vi "filter_chebyshev.vi"() -> ()   [LabVIEW 2014]
uses:
  <vilib>/addons/Digital Filter Design/_Objects.llb/DFD Phase Setting.ctl
  <vilib>/addons/Digital Filter Design/Analysis.llb/DFD Plot Freq Response (Linear-Spaced).vi
  <vilib>/addons/Digital Filter Design/NI_DigFilterLicensed.lvlib
panel:
  in  "Ripple":dbl(slide)=1.0 min=1.0 scale=0.0..10.0
  in  "High Cutoff Frequency":dbl(knob)=10.0 min=10.0 scale=0.0..1000.0
  in  "Low Cutoff Frequency":dbl(knob)=1.0 min=1.0 scale=0.0..1000.0
  in  "Scale":bool
  in  "Sampling Rate":dbl=1000.0 min=1000.0
  out "magnitude response":cluster{"f0":dbl, "df":dbl, "values":dbl[]}[](graph)
  out "phase response":cluster{"f0":dbl, "df":dbl, "values":dbl[]}[](graph)
  in  "Order":dbl=1.0 min=1.0
  in  "Filter Type":u16(ring) items=["Lowpass", "Highpass", "Bandpass", "Bandstop"]
  in  "stop":bool
  # "IIR Chebyshev Filters"
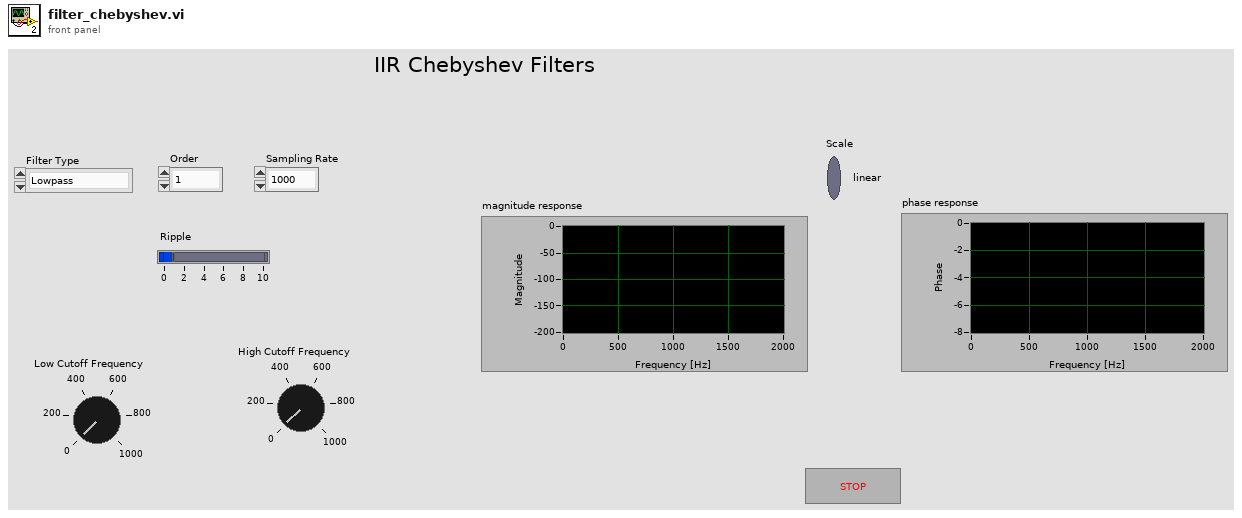
[diagram p1: front panel]
types:
  T1 = typedef "NI_DigFilterLicensed.lvlib/DFD Phase Setting.ctl" = cluster{"unwrap? (F)":bool, "degree? (F)":bool}
  T2 = typedef "NI_DigFilterLicensed.lvlib/DFD Filter Obj.ctl" = cluster{"mSRate_Fs":dbl, "mSRate_Version":string, "mSRate_Comments":string, "mSRate_OrgCoef":T3, "mSRate_CurCoef":T3, "mSRate_Quantized?":bool, "mSRate_QCoef":T3, "mSRate_QSettings":T5[], "mSRate_Order":i32, "mSRate_Scaling":cluster{"mSRate_ScaleByPowerOf2?":bool, "mSRate_ScaleType":T7}}
  T3 = typedef "NI_DigFilterLicensed.lvlib/DFD Filter Coef.ctl" = cluster{"type":T4, "gain":dbl, "coef a (k)":dbl[], "coef b (v)":dbl[]}
  T4 = typedef "NI_DigFilterLicensed.lvlib/DFD Filter Structure Type Selector.ctl" = enum16{"Undefined", "FIR Direct Form", "FIR Direct Form Transposed", "FIR Symmetric", "FIR Antisymmetric", "IIR Direct Form I", "IIR Direct Form I Transposed", "IIR Direct Form II", "IIR Direct Form II Transposed", "IIR Cascaded Second Order Sections Form I", "IIR Cascaded Second Order Sections Form I Transposed", "IIR Cascaded Second Order Sections Form II", "IIR Cascaded Second Order Sections Form II Transposed", "Lattice Allpass (basic sections)", "Lattice Allpass (one multiplier sections)", "Lattice Allpass (normalized sections)", "Lattice AR (basic sections)", "Lattice AR (one multiplier sections)", "Lattice AR (normalized sections)", "Lattice MA (minimum phase)", "Lattice MA (maximum phase)", "Lattice ARMA (basic sections)", "Lattice ARMA (one multiplier sections)", "Lattice ARMA (normalized sections)"}
  T5 = typedef "NI_DigFilterLicensed.lvlib/dfd_Internal Quantization Settings.ctl" = cluster{"source":T6, "wl":i16, "iwl":i16, "overflow mode":enum16{"Saturation", "Wrap"}, "rounding mode":enum16{"Nearest", "Truncation"}, "signed?":bool}
  T6 = typedef "NI_DigFilterLicensed.lvlib/dfd_Internal Quantization Srcs.ctl" = u16
  T7 = typedef "NI_DigFilterLicensed.lvlib/DFD Coef Norm Type.ctl" = enum16{"No Norm", "Time Domain 1-Norm", "Time Domain 2-Norm", "Time Domain Inf-Norm"}
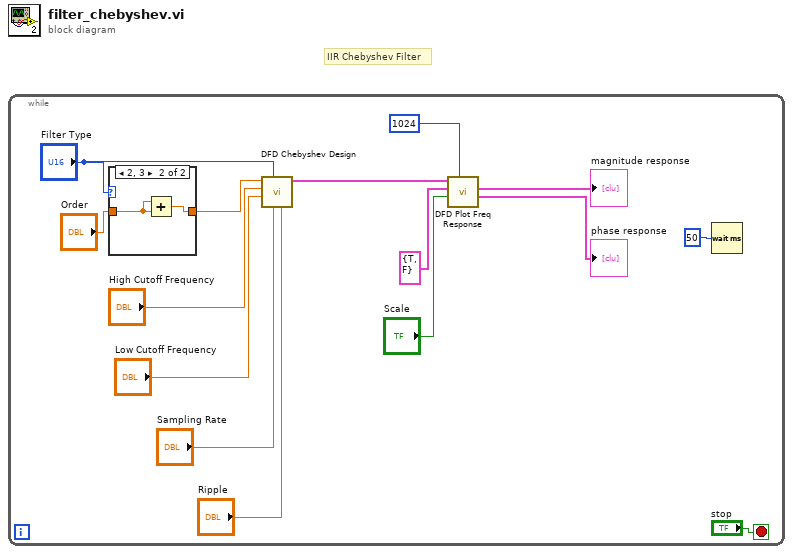
[diagram p0: block diagram]
diagram:
  # "IIR Chebyshev Filter"
  n1 = while {
    stop <- "stop" stop-if-true
    n2 = case shown="2, 3" "Filter Type" {
      tunnel: "Order" -> [w16 w17]
      tunnel: [w16 w18] -> w11
      frame 0, 1, Default {
      }
      frame 2, 3 {
        n3 = Add(x=w17, y=w17) -> (x+y=w18:dbl)
      }
    }
    n4 = call <vilib>:"DFD Chebyshev Design.vi"("passband ripple [dB]"="Ripple", "fs [Hz]"="Sampling Rate", "filter type"="Filter Type", "low cutoff freq [Hz]"="Low Cutoff Frequency", "high cutoff freq [Hz]"="High Cutoff Frequency", "order"=w11) -> ("filter out"=w13:T2)  [unwired: 1 in, 4 out]
    n5 = call-poly <vilib>:"DFD Plot Freq Response.vi"("# freq bins"=1024 ("# freq bins (auto)"), "dB on? (T)"="Scale", "phase view"=T1 {"unwrap? (F)"=TRUE, "degree? (F)"=FALSE}, "filter in"=w13) -> ("phase response"=→"phase response":cluster{"f0":dbl, "df":dbl, "values":dbl[]}[], "magnitude response"=→"magnitude response":cluster{"f0":dbl, "df":dbl, "values":dbl[]}[])  [unwired: 4 in, 2 out]
    n6 = Wait (ms)(milliseconds to wait=u32 50) -> ()  [unwired: 1 out]
  }
